vi "SetLayeredWindowAttributs.vi"(8 "error in (no error)":errorcluster, 10 "Color":u32(colorbox)=16777225, 11 "hw":u32) -> (0 "error out":errorcluster, 3 "hw 2":u32)   [LabVIEW 2019]
uses:
  user32.dll
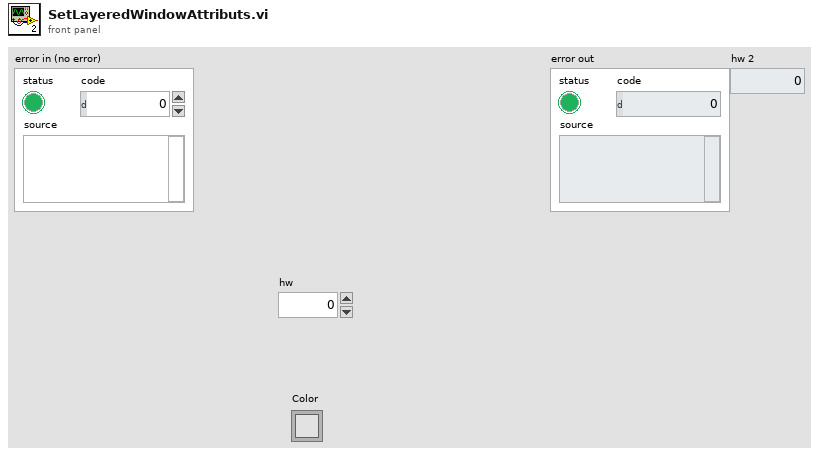
[diagram p1: front panel]
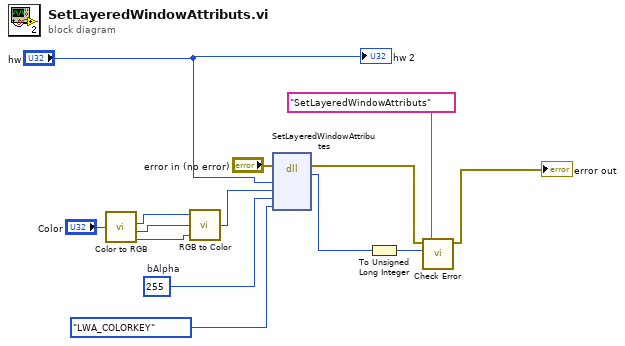
[diagram p0: block diagram]
diagram:
  w14 = u8 255  # bAlpha
  n1 = call <vilib>:"Color to RGB.vi"("Color"="Color") -> ("R"=w13:u8, "G"=w12:u8, "B"=w11:u8)  [unwired: 1 out]
  n2 = call <vilib>:"RGB to Color.vi"("B"=w11, "G"=w12, "R"=w13) -> ("Color"=w2:u32)
  n3 = dll-call lib="user32.dll" fn="SetLayeredWindowAttributes" label="SetLayeredWindowAttributs"(error in="error in (no error)", "handle"="hw", "crkey"=w2, "bAlpha"=w14, "dwFlags"=enum16{"NONE", "LWA_COLORKEY", "LWA_ALPHA"}."LWA_COLORKEY") -> (error out=w7:errorcluster, "return type"=w4:i32)  [unwired: 4 in, 3 out]
  n4 = To Unsigned Long Integer(number=w4) -> (unsigned 32bit integer=w3:u32)
  n5 = call "Check Error.vi"("Description"="SetLayeredWindowAttributs", "Return Code"=w3, "error in (no error)"=w7) -> ("error out"=→"error out":errorcluster)  [unwired: 8 in]
  "hw 2" <- "hw"
